vi "Initial Path Plot Sub_VI.vi"(10 "Motion Inputs":T4) -> (1 "Accel Array":dbl[](graph), 2 "Velocity Array":dbl[](graph), 3 "Displacement Array":dbl[](graph), 4 "V max (mm/s)":dbl, 5 "Motion Points":T2, 6 "Dist max (mm)":dbl, 7 "Motion Outputs":T3)   [LabVIEW 2017]
panel:
  out "Motion Planning Outputs":T1
  out "Waveform Chart":T2(graph)
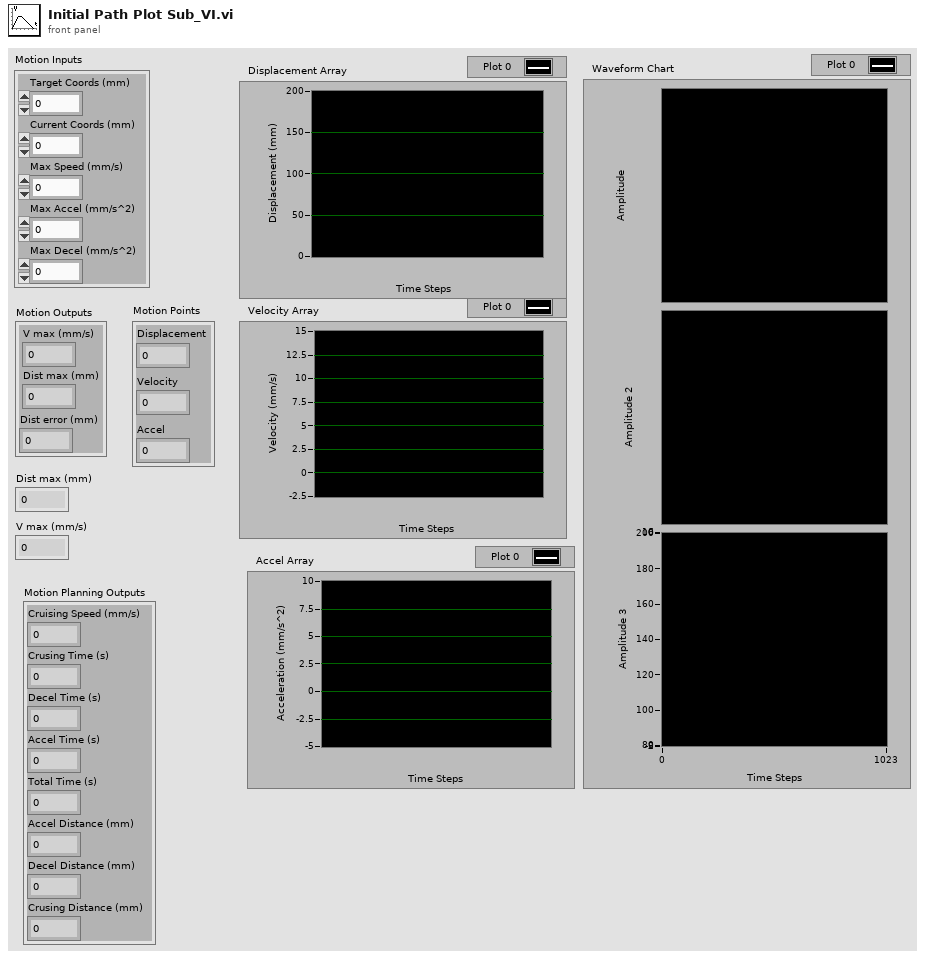
[diagram p1: front panel]
types:
  T1 = cluster{"Cruising Speed (mm/s)":dbl, "Crusing Time (s)":dbl, "Decel Time (s)":dbl, "Accel Time (s)":dbl, "Total Time (s)":dbl, "Accel Distance (mm)":dbl, "Decel Distance (mm)":dbl, "Crusing Distance (mm)":dbl}
  T2 = cluster{"Accel":dbl, "Velocity":dbl, "Displacement":dbl}
  T3 = cluster{"V max (mm/s)":dbl, "Dist max (mm)":dbl, "Dist error (mm)":dbl}
  T4 = cluster{"Target Coords (mm)":dbl, "Current Coords (mm)":dbl, "Max Speed (mm/s)":dbl, "Max Accel (mm/s^2)":dbl, "Max Decel (mm/s^2)":dbl}
  T5 = cluster{" Distance target (mm)":dbl, "Max Accel (mm/s^2)":dbl, "Max Decel (mm/s^2)":dbl, "Velocity Limit (mm/s) ":dbl, "Time step (s)":dbl}
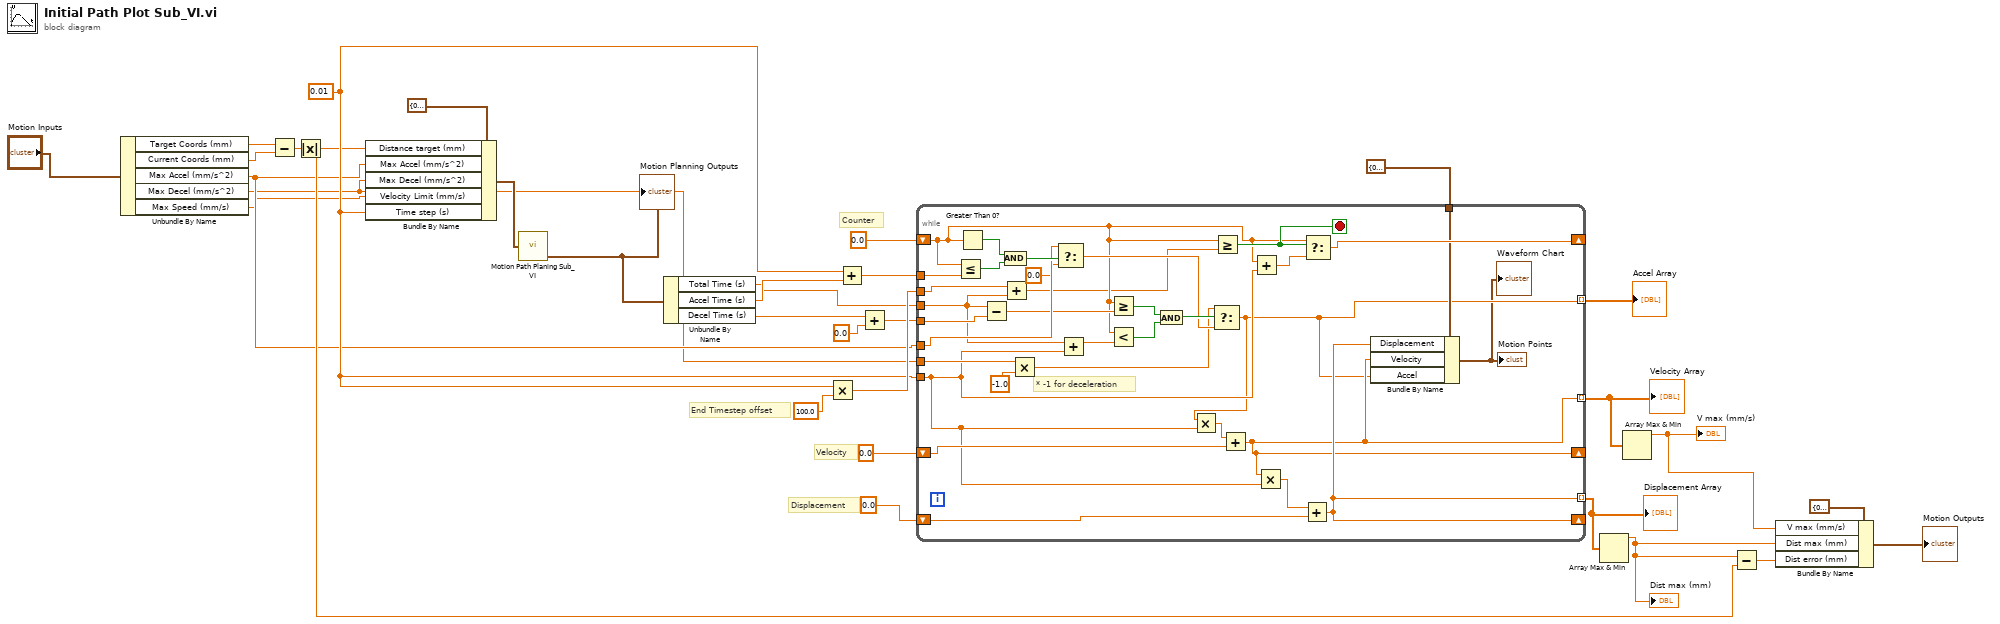
[diagram p0: block diagram]
diagram:
  w5 = 0.01 ("Time step (s)")
  # "End Timestep offset"
  # "Displacement"
  # "Velocity"
  # "Counter"
  n1 = Unbundle By Name("Motion Inputs") -> ("Target Coords (mm)"=w10:dbl, "Current Coords (mm)"=w9:dbl, "Max Accel (mm/s^2)"=w3:dbl, "Max Decel (mm/s^2)"=w2:dbl, "Max Speed (mm/s)"=w1:dbl)
  n2 = Subtract(x=w10, y=w9) -> (x-y=w29:dbl)
  n3 = Absolute Value(x=w29) -> (abs(x)=w4:dbl)
  n4 = Bundle By Name(cluster=T5 {" Distance target (mm)"=0.0, "Max Accel (mm/s^2)"=0.0, "Max Decel (mm/s^2)"=0.0, "Velocity Limit (mm/s) "=0.0, "Time step (s)"=0.0} ("Motion Planning Inputs"), "Distance target (mm)"=w4, "Max Accel (mm/s^2)"=w3, "Max Decel (mm/s^2)"=w2, "Velocity Limit (mm/s)"=w1, "Time step (s)"=w5) -> (w6:T5)
  n5 = call "Motion Path Planing Sub_VI.vi"("Motion Planning Inputs"=w6) -> ("Motion Planning Outputs"=w11:T1)  [unwired: 4 in, 2 out]
  "Motion Planning Outputs" <- w11
  n6 = Unbundle By Name(w11) -> ("Total Time (s)"=w13:dbl, "Accel Time (s)"=w14:dbl, "Decel Time (s)"=w12:dbl)
  n7 = Multiply(x=w5, y=100.0) -> (x*y=w27:dbl)
  n8 = Add(x=w5, y=w14) -> (x+y=w23:dbl)
  n9 = Add(x=w12, y=0.0) -> (x+y=w24:dbl)
  n10 = while {
    shift-right: [w43] -> _
    shift-left: 0.0 -> [w42]
    tunnel: w23 -> [w65]
    tunnel: w3 -> [w61]
    tunnel: w13 -> [w53]
    tunnel: w24 -> [w58]
    tunnel: [w34] -> w19 mode=indexing
    tunnel: w2 -> [w45]
    shift-right: [w35] -> _
    shift-left: 0.0 -> [w50]
    shift-right: [w37] -> _
    shift-left: 0.0 -> [w48]
    tunnel: [w35] -> w28 mode=indexing
    tunnel: [w37] -> w18 mode=indexing
    tunnel: w5 -> [w40]
    tunnel: w27 -> [w38]
    tunnel: T2 {"Accel"=0.0, "Velocity"=0.0, "Displacement"=0.0} ("Motion Points 2") -> [w36]
    stop <- w51 stop-if-true
    # "* -1 for deceleration"
    n11 = Less Or Equal?(x=w42, y=w65) -> (x <= y?=w63:bool)
    n12 = Greater Than 0?(x=w42) -> (x > 0?=w64:bool)
    n13 = Subtract(x=w53, y=w58) -> (x-y=w59:dbl)
    n14 = And(x=w64, y=w63) -> (x .and. y?=w62:bool)
    n15 = Add(x=w38, y=w53) -> (x+y=w39:dbl)
    n16 = Multiply(x=w45, y=-1.0 ("x")) -> (x*y=w46:dbl)
    n17 = Select(t=w61, s=w62, f=0.0) -> (s? t:f=w54:dbl)
    n18 = Add(x=w53, y=w40) -> (x+y=w41:dbl)
    n19 = Greater Or Equal?(x=w42, y=w59) -> (x >= y?=w57:bool)
    n20 = Less?(x=w42, y=w41) -> (x < y?=w56:bool)
    n21 = And(x=w57, y=w56) -> (x .and. y?=w55:bool)
    n22 = Select(t=w46, s=w55, f=w54) -> (s? t:f=w34:dbl)
    n23 = Multiply(x=w34, y=w40) -> (x*y=w49:dbl)
    n24 = Greater Or Equal?(x=w42, y=w39) -> (x >= y?=w51:bool)
    n25 = Add(x=w49, y=w50) -> (x+y=w35:dbl)
    n26 = Add(x=w42, y=w40) -> (x+y=w52:dbl)
    n27 = Multiply(x=w35, y=w40) -> (x*y=w47:dbl)
    n28 = Add(x=w47, y=w48) -> (x+y=w37:dbl)
    n29 = Select(t=w42, s=w51, f=w52) -> (s? t:f=w43:dbl)
    n30 = Bundle By Name(cluster=w36, "Displacement"=w37, "Velocity"=w35, "Accel"=w34) -> (→"Motion Points" →"Waveform Chart":T2)
  }
  "Accel Array" <- w19
  "Velocity Array" <- w28
  "Displacement Array" <- w18
  n31 = Array Max & Min(array=w18) -> (max value=w16:dbl)  [unwired: 3 out]
  "Dist max (mm)" <- w16
  n32 = Array Max & Min(array=w28) -> (max value=w15:dbl)  [unwired: 3 out]
  "V max (mm/s)" <- w15
  n33 = Subtract(x=w16, y=w4) -> (x-y=w31:dbl)
  n34 = Bundle By Name(cluster=T3 {"V max (mm/s)"=0.0, "Dist max (mm)"=0.0, "Dist error (mm)"=0.0} ("Motion Outputs 2"), "V max (mm/s)"=w15, "Dist max (mm)"=w16, "Dist error (mm)"=w31) -> (→"Motion Outputs":T3)
